vi "Get Next Windows Message.vi"(0 "win msg queue":T2, 1 "error in (no error)":errorcluster) -> (2 "win msg queue out":T2, 3 "Message":T1, 4 "Sent":bool, 5 "error out":errorcluster)   [LabVIEW 2010, in "Windows messages for Labview (32 and 64).lvlib"]
doc: "Removes the next message from the windows message queue and returns it. This should only be used after a call to Windows Message Queue Size.vi is used to determine how many messages are available in the queue.\n\nParameters:\nwin msg queue: the queue from which to remove the message.\n\nMessage: the message returned. The cluster is of the same format as the Windows MSG structure and contains the following information:\n hWnd: the handle of the window to which the message was posted\n message: the message\n wParam: the wParam parameter. Specific meaning depends on message.\n lParam: the lParam parameter. Specific meaning depends on message.\n time: system time at which the message was posted\n point: point cluster contain mouse positon in screen \n coordinates at the time of message posting\n\nSent: returns true if the message was sent to the window (via a call to SendMessage) or false if the message was posted (via PostMessage). Note: messages that are sent will not have valid time or point parameters.\n\nErrors:\n6751: Not a valid windows message queue.\n6752: No elements in queue."
uses:
  Windows messages for Labview (32 and 64).lvlib
  windows message x64.ctl
  Windows Messages for LabVIEW_64.dll
  windows message x32.ctl
  Windows Messages for LabVIEW_32.dll
  Win Msg Queue RefNum.ctl
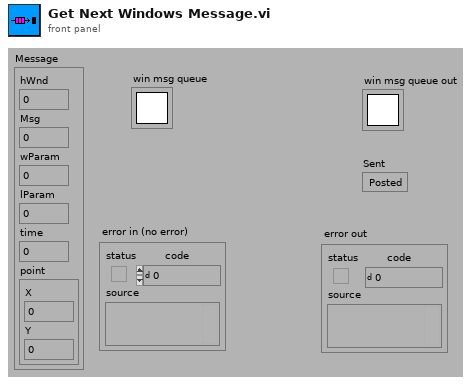
[diagram p1: front panel]
types:
  T1 = typedef "Windows messages for Labview (32 and 64).lvlib/windows message x64.ctl" = cluster{"hWnd":u64, "Msg":u32, "wParam":u64, "lParam":i32, "time":u32, "point":cluster{"X":i32, "Y":i32}}
  T2 = typedef "Windows messages for Labview (32 and 64).lvlib/Win Msg Queue RefNum.ctl" = refnum<k1>
  T3 = cluster{"hWnd":u32, "Msg":u32, "wParam":u32, "lParam":i32, "time":u32, "point":cluster{"X":i32, "Y":i32}}
  T4 = typedef "Windows messages for Labview (32 and 64).lvlib/windows message x32.ctl" = cluster{"hWnd":u32, "Msg":u32, "wParam":u32, "lParam":i32, "time":u32, "point":cluster{"X":i32, "Y":i32}}
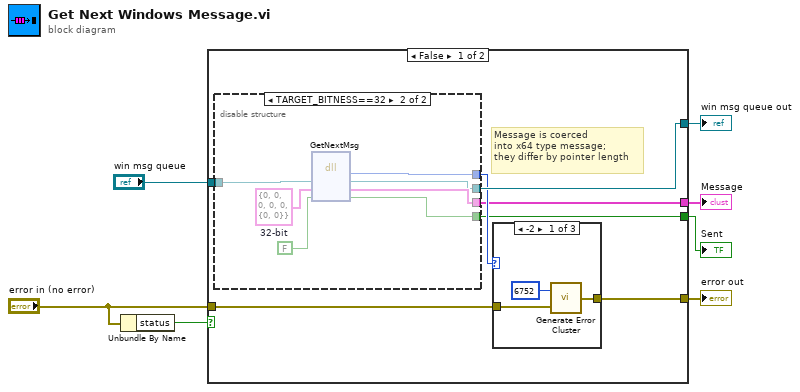
[diagram p0: block diagram]
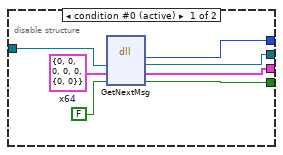
[diagram p2: hidden frame]
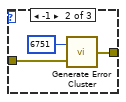
[diagram p3: hidden frame]
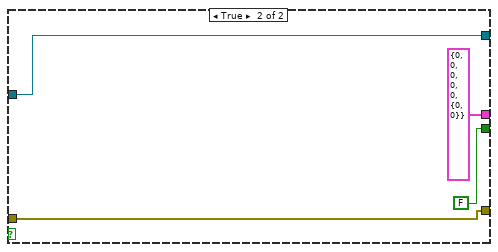
[diagram p5: hidden frame]
diagram:
  n1 = Unbundle By Name("error in (no error)") -> ("status"=w4:bool)
  n2 = case shown="False" w4 {
    tunnel: "win msg queue" -> [w12 w37]
    tunnel: [w9 T3 {"hWnd"=0, "Msg"=0, "wParam"=0, "lParam"=0, "time"=0, "point"={"X"=0, "Y"=0}} ("Input Value")] -> w1
    tunnel: "error in (no error)" -> [w14 w39]
    tunnel: [w13 w39] -> w5
    tunnel: [w11 w37] -> w3
    tunnel: [w8 FALSE] -> w2
    frame False {
      # "Message is coerced\ninto x64 type message;\nthey differ by pointer length"
      n3 = disable-structure shown="TARGET_BITNESS==32" {
        disable-tunnel: w12 -> [w20 w28]
        disable-tunnel: [w19 w23] -> w11
        disable-tunnel: [w18 w22] -> w10
        disable-tunnel: [w17 w25] -> w9
        disable-tunnel: [w15 w24] -> w8
        frame condition #0 (active) {
          w21 = T1 {"hWnd"=0, "Msg"=0, "wParam"=0, "lParam"=0, "time"=0, "point"={"X"=0, "Y"=0}}  # x64
          n4 = dll-call lib="P:/hagen/PDLM/API/Demos/LabVIEW/LabVIEW2017/_lib/Windows Messages for Labview/llb/Windows Messages for LabVIEW_64.dll" fn="GetNextMsg"("occurrence"=w20, "Msg"=w21, "postorsend"=FALSE) -> ("return type"=w18:i32, "occurrence"=w19:T2, "Msg"=w17:T1, "postorsend"=w15:bool)  [unwired: 3 in, 2 out]
        }
        frame condition #1 {
          w26 = T4 {"hWnd"=0, "Msg"=0, "wParam"=0, "lParam"=0, "time"=0, "point"={"X"=0, "Y"=0}}  # 32-bit
          n5 = dll-call lib="D:/labview_d/temp/Windows Messaging/Windows Messages for Labview/llb/Windows Messages for LabVIEW_32.dll" fn="GetNextMsg"("occurrence"=w28, "Msg"=w26, "postorsend"=FALSE) -> ("return type"=w22:i32, "occurrence"=w23:T2, "Msg"=w25:T4, "postorsend"=w24:bool)  [unwired: 3 in, 2 out]
        }
      }
      n6 = case shown="-2" w10 {
        tunnel: w14 -> [w30 w33 w35]
        tunnel: [w31 w34 w35] -> w13
        frame -2 {
          n7 = call "Generate Error Cluster.vi"("error in (no error)"=w30, "Error Code"=6752) -> ("error out"=w31:errorcluster)
        }
        frame -1 {
          n8 = call "Generate Error Cluster.vi"("error in (no error)"=w33, "Error Code"=6751) -> ("error out"=w34:errorcluster)
        }
        frame 1, Default {
        }
      }
    }
    frame True {
    }
  }
  "error out" <- w5
  "win msg queue out" <- w3
  "Sent" <- w2
  "Message" <- w1
